vi "Status Det.vi"(8 "error in (no error)":errorcluster, 10 "data":variant, 11 "Control-Client in":refnum<class "Control-Client.lvclass">) -> (0 "error out":errorcluster, 2 "error IO":errorcluster, 3 "Control-Client out":refnum<class "Control-Client.lvclass">)   [LabVIEW 2019, in "Control-Client.lvclass"]
uses:
  Control-Client.lvclass
  C:/Dev/TRANCON/Classes/GeneralFunctionality/GeneralFunctionality.lvclass
  dependecies/ControlsVIs/Clusters-def/Det-Reply-to-Connect-client.ctl
  dependecies/ControlsVIs/Clusters-def/Commands-CLIENT.ctl
  dependecies/ControlsVIs/Clusters-def/Message types.ctl
  dependecies/ControlsVIs/Clusters-def/SERVER-Commands.ctl
  dependecies/ControlsVIs/Clusters-def/Def_Vis_Update.ctl
  Control-Client.lvclass/Control-Client.ctl
  controls/Gauge_pump/Gauge_pump.xctl
  dependecies/XControls/CellsDL/ControlDL.xctl
  Detector/Detector.lvclass
  Message/Message.lvclass
  GeneralFunctionality/GeneralFunctionality.lvclass
  Control-Server/Control-Server.lvclass
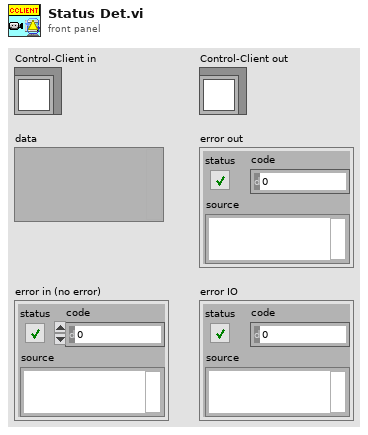
[diagram p1: front panel]
types:
  T1 = typedef "Control-Client.lvclass/Def_Vis_Update.ctl" = cluster{"Data":sgl[][], "timedelays":dbl[], "wavelength":dbl[]}
  T2 = typedef "Message types.ctl" = string
  T3 = typedef "Control-Server.lvclass/SERVER-Commands.ctl" = string
  T4 = typedef "Control-Client.lvclass/Commands-CLIENT.ctl" = string
  T5 = typedef "Detector.lvclass/Det-Reply-to-Connect-client.ctl" = cluster{"on/off":bool, "calibration":dbl[], "error":errorcluster}
  T6 = typedef "Control-Client.lvclass/Controls-with-permissions_CLIENT.ctl" = cluster{"Server ON/OFF":refnum<vi>, "Detector connect":refnum<vi>, "DL connect":refnum<vi>, "DAQmx connect":refnum<vi>, "All connect":refnum<vi>, "Start measurement":refnum<vi>, "Move Crystal":refnum<vi>, "Relay key heater":refnum<vi>, "Laser Shutter":refnum<vi>, "Accelerator Shutter":refnum<vi>, "Power":refnum<vi>, "Unlock":refnum<vi>, "RT":refnum<vi>, "Faraday Cup":refnum<vi>, "Osc connect":refnum<vi>, "ELYSE pulses":refnum<vi>, "Cells":refnum<vi>, "Pump":refnum<vi>, "# par point":refnum<vi>, "Alarm":refnum<vi>, "oscilloscopeRead":refnum<vi>, "WCM_state":refnum<vi>, "ControlDL":refnum<vi>}
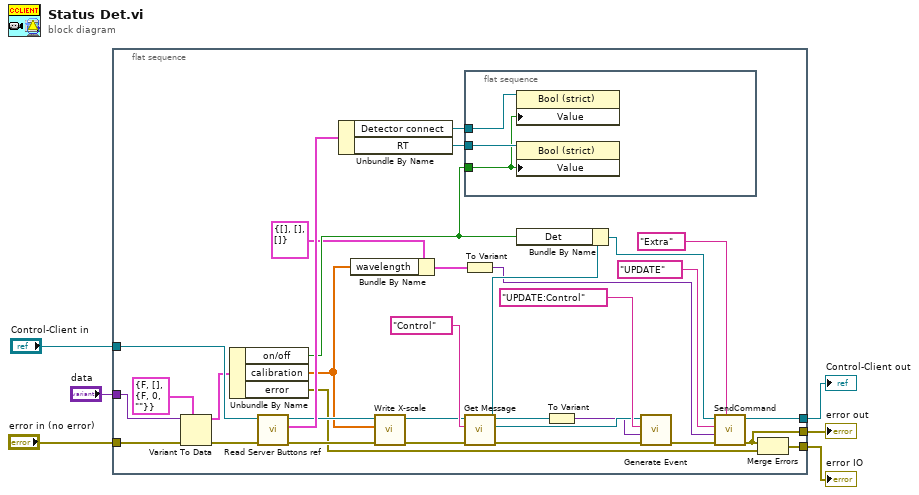
[diagram p0: block diagram]
diagram:
  n1 = flat-sequence {
    tunnel: "data" -> [w38]
    tunnel: "Control-Client in" -> [w37]
    tunnel: "error in (no error)" -> [w35]
    tunnel: [w8] -> w4
    tunnel: [w7] -> w5
    tunnel: [w20] -> w6
    frame #0 {
      n2 = Variant To Data(error in=w35, type=T5 {"on/off"=FALSE, "calibration"=[], "error"={"status"=FALSE, "code"=0, "source"=""}} ("Cluster"), Variant=w38) -> (data=w32:T5, error out=w36:errorcluster)
      n3 = Unbundle By Name(w32) -> ("on/off"=w18:bool, "calibration"=w13:dbl[], "error"=w21:errorcluster)
      n4 = call "Read Server Buttons ref.vi"("error in (no error)"=w36, "Control-Client in"=w37) -> ("error out"=w22:errorcluster, "Server Buttons ref"=w34:T6, "Control-Client out"=w23:refnum<class "Control-Client.lvclass">)  [unwired: 7 in]
      n5 = Unbundle By Name(w34) -> ("Detector connect"=w33:refnum<vi>, "RT"=w19:refnum<vi>)
      n6 = Bundle By Name(cluster=T1 {"Data"=[], "timedelays"=[], "wavelength"=[]}, "wavelength"=w13) -> (w11:T1)
      n7 = call "Write X-scale.vi"("error in (no error)"=w22, "X-scale"=w13, "Control-Client in"=w23) -> ("error out"=w25:errorcluster, "Control-Client out"=w24:refnum<class "Control-Client.lvclass">)  [unwired: 7 in]
      n8 = flat-sequence {
        tunnel: w33 -> [w41]
        tunnel: w19 -> [w40]
        tunnel: w18 -> [w39]
        frame #0 {
          n9 = property class="Bool (strict)"(reference=w41, "Value"=w39) -> ()  [unwired: 1 in, 2 out]
          n10 = property class="Bool (strict)"(reference=w40, "Value"=w39) -> ()  [unwired: 1 in, 2 out]
        }
      }
      n11 = To Variant(anything=w11) -> (Variant=w10:variant)
      n12 = call "Get Message.vi"("error in (no error)"=w25, "Message type"=T2 "Control", "GeneralFunctionality en entrée"=w24) -> ("error out"=w27:errorcluster, "Message.lvclass"=w29:refnum<class "Message.lvclass">, "GeneralFunctionality en sortie"=w17:refnum<class "Control-Client.lvclass">)  [unwired: 6 in]
      n13 = Bundle By Name(cluster=w17, "Det"=w18) -> (w9:refnum<class "Control-Client.lvclass">)
      n14 = To Variant(anything=w17) -> (Variant=w26:variant)
      n15 = call "Generate Event.vi"("error in (no error)"=w27, "Data"=w26, "Command"=T4 "UPDATE:Control" ("Commands-Client"), "Message en entrée"=w29) -> ("error out"=w12:errorcluster)  [unwired: 6 in, 1 out]
      n16 = call "SendCommand.vi"("Message type"=T2 "Extra", "error in (no error)"=w12, "data"=w10, "Command"=T3 "UPDATE" ("Commands"), "Control-Client in"=w9) -> ("error out"=w7:errorcluster, "Control-Client out"=w8:refnum<class "Control-Client.lvclass">)  [unwired: 5 in]
      n17 = Merge Errors(w7, w21) -> (w20:errorcluster)
    }
  }
  "error IO" <- w6
  "error out" <- w5
  "Control-Client out" <- w4
